vi "Calculate avg5.vi"(8 "error in (no error)":errorcluster, 9 "Number of values for avg":i32=4, 10 "New Values":dbl[][](array[numeric]), 11 "Old Values":dbl[][][](array[numeric])) -> (0 "error out":errorcluster, 2 "New Values":dbl[][](array[numeric]), 3 "Contencated Values":dbl[][][](array[numeric]))   [LabVIEW 2017, in "Akwizycja.lvlib"]
uses:
  Akwizycja.lvlib
panel:
  out "cluster":cluster{"[0]":i32, "[1]":i32, "[2]":i32}
  out "x/y":dbl[][](array[numeric])
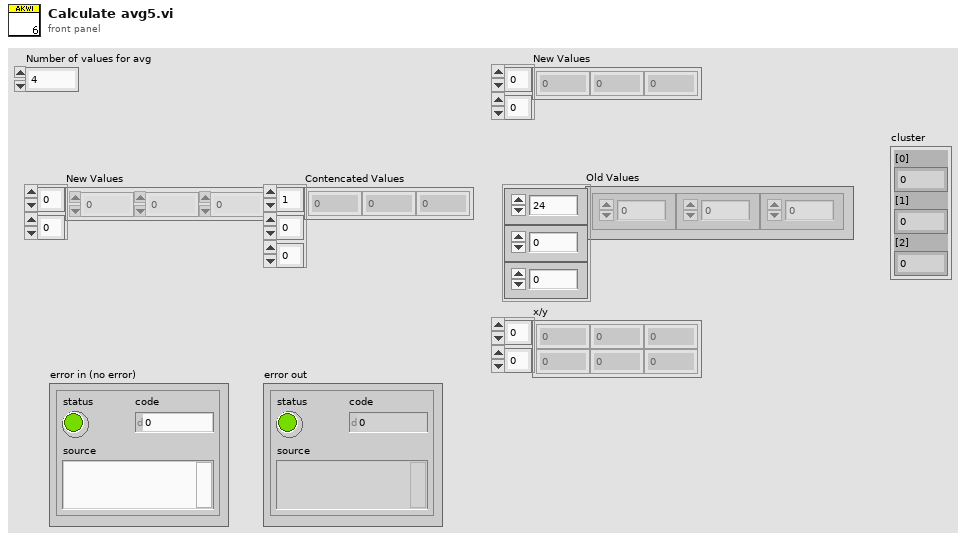
[diagram p1: front panel]
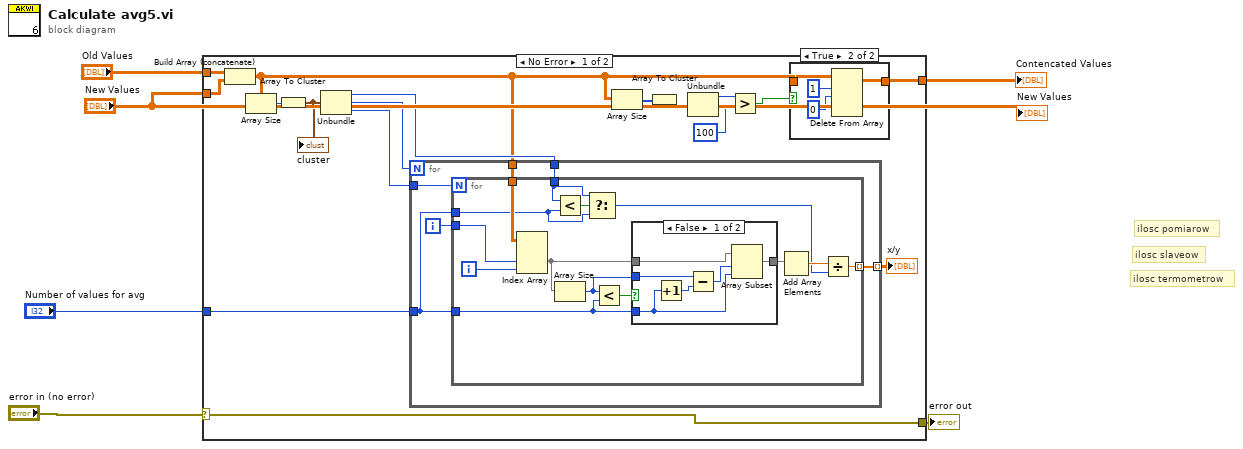
[diagram p0: block diagram]
diagram:
  # "ilosc pomiarow"
  # "ilosc slaveow"
  # "ilosc termometrow"
  n1 = case shown="No Error" "error in (no error)" {
    selector: "error in (no error)" -> [w23 w57]
    tunnel: [w23 w57] -> w4
    tunnel: "New Values" -> [w21 _]
    tunnel: "Old Values" -> [w22 w56]
    tunnel: [w10 w56] -> w2
    tunnel: "Number of values for avg" -> [w14 _]
    frame No Error {
      n2 = Build Array (concatenate)(w22, w21) -> (w11:dbl[][][])
      n3 = Array Size(array=w11) -> (size(s)=w20:i32[])
      n4 = Array To Cluster(array=w20) -> (cluster=w19:cluster{"[0]":i32, "[1]":i32, "[2]":i32})
      "cluster" <- w19
      n5 = Unbundle(w19) -> ("[0]"=w16:i32, "[1]"=w18:i32, "[2]"=w17:i32)
      n6 = for {
        N: w18 -> [_]
        tunnel: w17 -> [w34]
        tunnel: w16 -> [w33]
        tunnel: w11 -> [w32]
        tunnel: [w30] -> w15 mode=indexing
        tunnel: w14 -> [w29]
        i -> [w31]
        n7 = for {
          N: w34 -> [_]
          tunnel: w33 -> [w46]
          tunnel: w32 -> [w47]
          tunnel: w31 -> [w45]
          tunnel: [w41] -> w30 mode=indexing
          tunnel: w29 -> [w36]
          tunnel: w29 -> [w35]
          i -> [w44]
          n8 = Index Array(array=w47, index (dim 1)=w45, index (dim 2)=w44) -> (element=w39:dbl[])  [unwired: 1 in]
          n9 = Less?(x=w46, y=w35) -> (x < y?=w48:bool)
          n10 = Array Size(array=w39) -> (size(s)=w37:i32)
          n11 = Select(t=w46, s=w48, f=w35) -> (s? t:f=w42:i32)
          n12 = Less?(x=w37, y=w36) -> (x < y?=w40:bool)
          n13 = case shown="False" w40 {
            tunnel: w39 -> [w53 w55]
            tunnel: [w54 w55] -> w38
            tunnel: w37 -> [w52 _]
            tunnel: w36 -> [w49 _]
            frame False {
              n14 = Increment(x=w49) -> (x+1=w50:i32)
              n15 = Subtract(x=w52, y=w50) -> (x-y=w51:i32)
              n16 = Array Subset(array=w53, index=w51, length=w49) -> (w54:dbl[])
            }
            frame True {
            }
          }
          n17 = Add Array Elements(numeric array=w38) -> (sum=w43:dbl)
          n18 = Divide(x=w43, y=w42) -> (x/y=w41:dbl)
        }
      }
      "x/y" <- w15
      n19 = Array Size(array=w11) -> (size(s)=w13:i32[])
      n20 = Array To Cluster(array=w13) -> (cluster=w12:cluster{"[0]":i32, "[1]":i32, "[2]":i32})
      n21 = Unbundle(w12) -> ("[0]"=w9:i32)  [unwired: 2 out]
      n22 = Greater?(x=w9, y=100) -> (0:w7:bool)
      n23 = case shown="True" w7 {
        tunnel: w11 -> [w24 w27]
        tunnel: [w24 w26] -> w10
        frame False {
        }
        frame True {
          n24 = Delete From Array(array=w27, length=1, index (dim 0)=0 ("index (page)")) -> (array with subset deleted=w26:dbl[][][])  [unwired: 2 in, 1 out]
        }
      }
    }
    frame Error {
    }
  }
  "error out" <- w4
  "Contencated Values" <- w2
  "New Values" <- "New Values"
